vi "readSetDuration.vi"(6 "loop delay":dbl, 7 "Reading Option (0: Latest)":i32, 8 "error in (no error)":errorcluster, 9 "Electrometer in":refnum<class "Electrometer.lvclass">, 10 "duration":dbl, 11 "ReadyState in":refnum<class "ReadyState.lvclass">) -> (0 "error out":errorcluster, 1 "Electrometer out":refnum<class "Electrometer.lvclass">, 2 "results":dbl[](array[numeric]), 3 "ReadyState out":refnum<class "ReadyState.lvclass">)   [LabVIEW 2016, in "ReadyState.lvclass"]
uses:
  ReadyState.lvclass
  Electrometer.lvclass
panel:
  out "local stop":bool
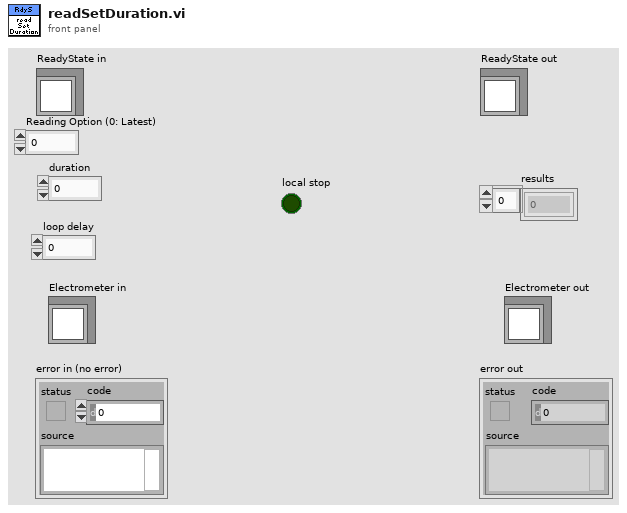
[diagram p1: front panel]
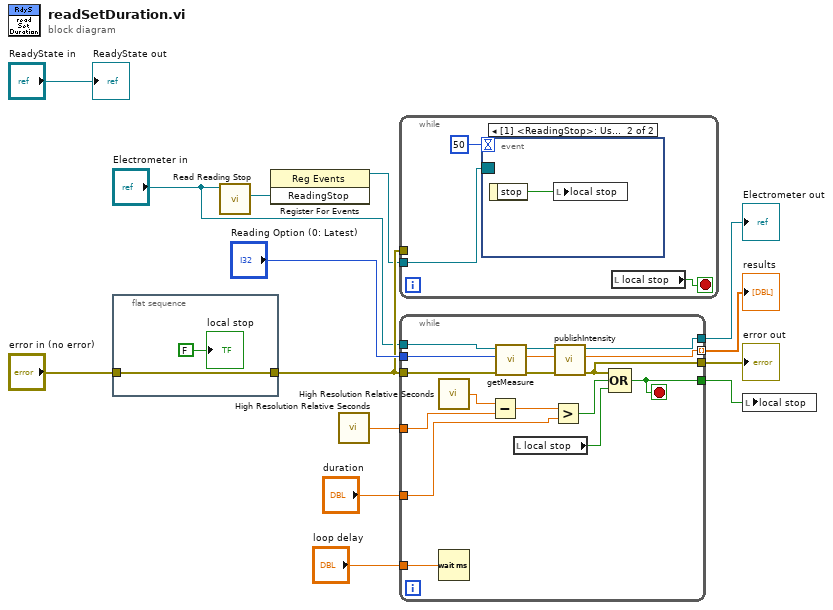
[diagram p0: block diagram]
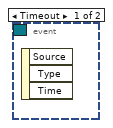
[diagram p2: hidden frame]
diagram:
  n1 = flat-sequence {
    tunnel: "error in (no error)" -> [w16]
    tunnel: [w16] -> w5
    frame #0 {
      "local stop" <- FALSE ("local stop")
    }
  }
  n2 = call-dynamic "Read Reading Stop.vi"("Electrometer in"="Electrometer in") -> ("ReadingStop"=w2:refnum<user-event>)  [unwired: 8 in, 2 out]
  n3 = register-events(w2) -> (reference out=w4:refnum<event-registration>)  [unwired: 2 in, 1 out]
  n4 = call <vilib>:"High Resolution Relative Seconds.vi"() -> ("relative seconds"=w8:dbl)
  n5 = while {
    tunnel: w4 -> [w18]
    tunnel: w5 -> [_]
    stop <- w19 stop-if-true
    n6 = event shown="[1] <ReadingStop>: User Event" {
      selector: w18 -> [_ _]
      dyn-events: _ -> [_ _]
      timeout: 50 -> [_ _]
      event Timeout {
        n7 = event-data() -> ()  [unwired: 1 in, 3 out]
      }
      event User Event {
        n8 = event-data() -> ("stop"=w20:bool)  [unwired: 1 in]
        n9 = local write "local stop"(w20) -> ()
      }
    }
    n10 = local read "local stop"() -> (w19:bool)
  }
  n11 = while {
    tunnel: w5 -> [w37]
    tunnel: "Electrometer in" -> [w27]
    tunnel: "loop delay" -> [w36]
    tunnel: [w21] -> w12 mode=indexing
    tunnel: [w22] -> w11
    tunnel: "Reading Option (0: Latest)" -> [w35]
    tunnel: "duration" -> [w34]
    tunnel: w8 -> [w31]
    tunnel: [w28] -> w6
    tunnel: [w23] -> w1
    stop <- w28 stop-if-true
    n12 = call <vilib>:"High Resolution Relative Seconds.vi"() -> ("relative seconds"=w32:dbl)
    n13 = Wait (ms)(milliseconds to wait=w36) -> ()  [unwired: 1 out]
    n14 = Subtract(x=w32, y=w31) -> (x-y=w33:dbl)
    n15 = call-dynamic "getMeasure.vi"("error in (no error)"=w37, "Reading Option (0: Latest)"=w35, "Electrometer in"=w27) -> ("error out"=w26:errorcluster, "Measure"=w24:dbl, "Electrometer out"=w25:refnum<class "Electrometer.lvclass">)  [unwired: 6 in]
    n16 = local read "local stop"() -> (w29:bool)
    n17 = Greater?(x=w33, y=w34) -> (0:w30:bool)
    n18 = call-dynamic "publishIntensity.vi"("error in (no error)"=w26, "Intensity"=w24, "Electrometer in"=w25) -> ("error out"=w23:errorcluster, "Intensity out"=w21:dbl, "Electrometer out"=w22:refnum<class "Electrometer.lvclass">)  [unwired: 6 in]
    n19 = Compound Arithmetic op=OR(w23, w30, w29) -> (w28:bool)
  }
  "error out" <- w1
  "Electrometer out" <- w11
  "results" <- w12
  n20 = local write "local stop"(w6) -> ()
  "ReadyState out" <- "ReadyState in"
